vi "Read Address.vi"(11 "Event Transport in":refnum<class "Event Transport.lvclass">) -> (2 "Address":refnum<data-value>)   [LabVIEW 2025, in "jettl.lvlib" / "Event Transport.lvlib" / "Event Transport.lvclass"]
uses:
  Event Transport.lvclass
  Event Transport.lvclass/Event Transport.ctl
  Msg/Msg.lvclass
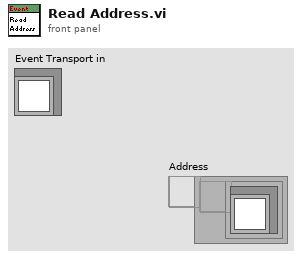
[diagram p1: front panel]
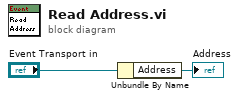
[diagram p0: block diagram]
diagram:
  n1 = Unbundle By Name("Event Transport in") -> ("Address"=→"Address":refnum<data-value>)
